vi "Run Simulated Demonstration.vi"() -> ()   [LabVIEW 2017]
doc: "Run a demonstration using a device driver, with the data shared across a local network.\n\nUses a configurable GUI, with multiple tabs and active plots.\n\nNote: the simulation does not make a connection to the DTACQ device, and uses random noise as the dataset."
uses:
  GUI/Plots/Plot Data - Main GUI.vi
  DTACQ - Network Enabled Device Driver.lvlib
  GUI/Plots/DTacq Plot Display Library.lvlib
panel:
  in  "Start Button":bool
  # "Simulation"
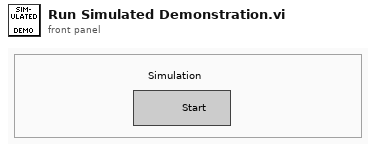
[diagram p1: front panel]
types:
  T1 = enum32{"Invalid", "Standard", "Closed", "Hidden", "Minimized", "Maximized"}
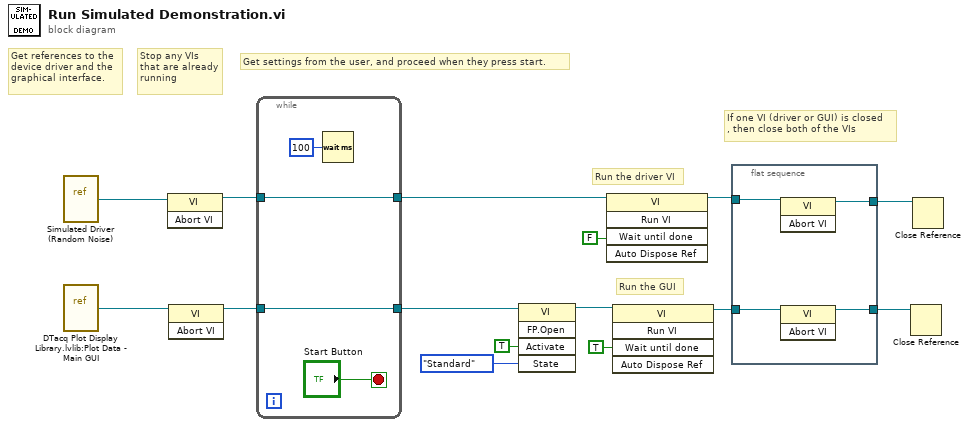
[diagram p0: block diagram]
diagram:
  # "If one VI (driver or GUI) is closed\n, then close both of the VIs"
  # "Run the GUI"
  # "Run the driver VI"
  # "Get settings from the user, and proceed when they press start."
  # "Stop any VIs\nthat are already\nrunning"
  # "Get references to the\ndevice driver and the\ngraphical interface."
  n1 = vi-ref "Simulated Driver (Random Noise).vi"() -> (w12:refnum<vi>)
  n2 = vi-ref "DTacq Plot Display Library.lvlib:Plot Data - Main GUI.vi"() -> (w11:refnum<vi>)
  n3 = invoke class="VI" method="Abort VI"(reference=w12) -> (reference out=w2:refnum<vi>)  [unwired: 2 in, 2 out]
  n4 = invoke class="VI" method="Abort VI"(reference=w11) -> (reference out=w4:refnum<vi>)  [unwired: 2 in, 2 out]
  n5 = while {
    tunnel: w4 -> [w18]
    tunnel: [w18] -> w3
    tunnel: w2 -> [w17]
    tunnel: [w17] -> w1
    stop <- "Start Button" stop-if-true
    n6 = Wait (ms)(milliseconds to wait=u32 100) -> ()  [unwired: 1 out]
  }
  n7 = invoke class="VI" method="FP.Open"(reference=w3, "Activate"=TRUE ("Activate?"), "State"=T1."Standard") -> (reference out=w10:refnum<vi>)  [unwired: 2 in, 4 out]
  n8 = invoke class="VI" method="Run VI"(reference=w1, "Wait until done"=FALSE ("Wait Until Done")) -> (reference out=w8:refnum<vi>)  [unwired: 3 in, 4 out]
  n9 = invoke class="VI" method="Run VI"(reference=w10, "Wait until done"=TRUE ("Wait Until Done")) -> (reference out=w7:refnum<vi>)  [unwired: 3 in, 4 out]
  n10 = flat-sequence {
    tunnel: w8 -> [w23]
    tunnel: w7 -> [w22]
    tunnel: [w21] -> w6
    tunnel: [w20] -> w5
    frame #0 {
      n11 = invoke class="VI" method="Abort VI"(reference=w23) -> (reference out=w20:refnum<vi>)  [unwired: 2 in, 2 out]
      n12 = invoke class="VI" method="Abort VI"(reference=w22) -> (reference out=w21:refnum<vi>)  [unwired: 2 in, 2 out]
    }
  }
  n13 = Close Reference(reference=w6) -> ()  [unwired: 1 in, 1 out]
  n14 = Close Reference(reference=w5) -> ()  [unwired: 1 in, 1 out]
